vi "Lockin-4461_Multiple Inputs and Outputs_KH_functional_global_waveform_2_2.vi"(8 "stop":bool) -> ()   [LabVIEW 2013]
uses:
  <vilib>/Analysis/4window.llb/windowTd.ctl
  <vilib>/Analysis/3filter.llb/Filter Structure Type.ctl
  <vilib>/Analysis/baseanly.llb/Mean (DBL).vi
  <vilib>/DAQmx/write.llb/DAQmx Write (Analog 1D Wfm NChan NSamp).vi
  <vilib>/Analysis/2dsp.llb/Decimate (single shot).vi
  <vilib>/Analysis/2dsp.llb/Decimate (single shot, DBL).vi
  DAQ-Lockin-SubVI/Lock-in Globles Multiple Inputs and Outputs used with FGV.vi
  <vilib>/Utility/error.llb/Error Cluster From Error Code.vi
  <vilib>/DAQmx/miscellaneous.llb/DAQmx Fill In Error Info.vi
  <vilib>/measure/macond.llb/IIR Filter for N Chan.vi
  <vilib>/measure/maspectr.llb/FFT Power Spectrum and PSD for N Chan.vi
  <vilib>/Analysis/NI_AALBase.lvlib
  <vilib>/measure/NI_MAPro.lvlib
  <vilib>/measure/NI_MABase.lvlib
  <vilib>/Analysis/NI_AALPro.lvlib
panel:
  in  "IIR filter specifications":T1={"Topology"=enum."Butterworth", "Type"=enum."Lowpass", "Order"=1, "Lower Fc"=100.0, "Upper Fc"=200.0, "PB Ripple"=1.0, "SB Attenuation"=60.0} {"PB Ripple" format="%0.2f"; "SB Attenuation" format="%0.2f"; "Lower Fc" format="%0.2p"; "Upper Fc" format="%0.2p"}
  in  "Input Signals":i16(slide)=2 scale=1.0..20.0
  out "phase log":dbl[](array[numeric])=[0.0, 0.0, 0.0, 0.0, 0.0, 6.661338147750939e-16, 0.0, 1.9984014443252818e-15]
  in  "Tab Control 2":T2(tab)=enum."Lock-in Settings"
  in  "Auto control  max AI rate/ AI block size":bool=TRUE
  in  "AI Buffer Size (S)":i32=10
  in  "AI Block Size":i32=1000
  in  "AI Configuration":T3(array[cluster])=[{"AI.Coupling"=10050, "AI.Max"=10.0, "AI.Min"=-10.0, "Input physical channels"="PXI1Slot2/ai0:1"}, {"AI.Coupling"=10050, "AI.Max"=10.0, "AI.Min"=-10.0, "Input physical channels"="PXI1Slot3/ai0:1"}, {"AI.Coupling"=10050, "AI.Max"=10.0, "AI.Min"=-10.0, "Input physical channels"="PXI1Slot5/ai0:1"}, {"AI.Coupling"=10050, "AI.Max"=10.0, "AI.Min"=-10.0, "Input physical channels"="PXI1Slot6/ai0:1"}] {"AI.Coupling" items=["AC"=10045, "DC"=10050, "GND"=10066]}
  in  "AO Configuration":T4(array[cluster])=[{"Output physical channels"="PXI1Slot2/ao0:1", "AO. Max"=0.1, "AO.Min"=-0.1}, {"Output physical channels"="PXI1Slot3/ao0:1", "AO. Max"=0.25, "AO.Min"=-0.25}, {"Output physical channels"="PXI1Slot5/ao0:1", "AO. Max"=0.1, "AO.Min"=-0.1}, {"Output physical channels"="PXI1Slot6/ao0:1", "AO. Max"=0.1, "AO.Min"=-0.1}]
  in  "OSC Configuration":T5(array[cluster])=[[{"Signal Type"=enum."Sine Wave", "DC"=0.0, "Amplitude"=0.01, "frequency"=13.0, "Phase"=0.0}, {"Signal Type"=enum."Sine Wave", "DC"=0.0, "Amplitude"=0.0, "frequency"=13.0, "Phase"=0.0}], [{"Signal Type"=enum."Sine Wave", "DC"=0.0, "Amplitude"=0.0, "frequency"=13.0, "Phase"=0.0}, {"Signal Type"=enum."Sine Wave", "DC"=0.0, "Amplitude"=0.0, "frequency"=13.0, "Phase"=0.0}], [{"Signal Type"=enum."Sine Wave", "DC"=0.0, "Amplitude"=0.0, "frequency"=13.0, "Phase"=0.0}, {"Signal Type"=enum."Sine Wave", "DC"=0.0, "Amplitude"=0.0, "frequency"=13.0, "Phase"=0.0}], [{"Signal Type"=enum."Sine Wave", "DC"=0.0, "Amplitude"=0.0, "frequency"=13.0, "Phase"=0.0}, {"Signal Type"=enum."Sine Wave", "DC"=0.0, "Amplitude"=0.0, "frequency"=13.0, "Phase"=0.0}]] {"frequency" step=0.001 format="%.3p"; "Amplitude" format="%0.2p"; "DC" min=-0.99 max=0.99 format="%.2p"}
  in  "Phase&Tc":T6(array[cluster])=[{"Phase"=0.0, "Time constant"=0.5, "Set Tc"=FALSE, "Autophase"=FALSE, "Order"=0.0}, {"Phase"=0.0, "Time constant"=0.5, "Set Tc"=FALSE, "Autophase"=FALSE, "Order"=0.0}, {"Phase"=0.0, "Time constant"=0.5, "Set Tc"=FALSE, "Autophase"=FALSE, "Order"=0.0}, {"Phase"=0.0, "Time constant"=0.5, "Set Tc"=FALSE, "Autophase"=FALSE, "Order"=0.0}, {"Phase"=0.0, "Time constant"=0.5, "Set Tc"=FALSE, "Autophase"=FALSE, "Order"=0.0}, {"Phase"=0.0, "Time constant"=0.5, "Set Tc"=FALSE, "Autophase"=FALSE, "Order"=0.0}, {"Phase"=0.0, "Time constant"=0.5, "Set Tc"=FALSE, "Autophase"=FALSE, "Order"=0.0}, {"Phase"=0.0, "Time constant"=0.5, "Set Tc"=FALSE, "Autophase"=FALSE, "Order"=0.0}] {"Phase" min=0.0 max=360.0 scale=0.0..360.0}
  in  "Gain":dbl[](array[numeric])=[50000000.0, 50000000.0, 1.0, 1.0, 1.0, 1.0, 1.0, 1.0]
  in  "frequency":dbl=13.0
  out "max ai rate":i32=13000
  out "elapsed time":dbl=138.0
  in  "zero offset":bool
  in  "measure offset":bool
  in  "sample clock multiple (x*f)":i32=1000
  out "AI Rate":dbl=13000.0 format="%.2f"
  out "Display 2":string="-423.350804      n"
  out "Display 1":string="-104.244723      n"
  in  "Remote":bool
  in  "Display":u16(ring) items=["X and Y", "R and Theta"]
  out "Backlog":u8(slide) scale=0.0..100.0
  out "Sampling information":cluster{"Fs":dbl, "#s":dbl}[](array[cluster])=[{"Fs"=13000.0, "#s"=1000.0}]
  out "AO Task":refnum<k21>[](array[refnum])
  out "AI task":refnum<k21>[](array[refnum])
  in  "Tab Control":T7(tab)=enum."Input signals"
  out "Display X (or R) A":dbl[](graph)=[-6.767704118237299e-07, 1.3679095941982762e-06, -8.292119972514093e-07, 1.6081112063430916e-06, -6.48302849428553e-07, 3.3000787620994813e-07, 2.1826626593165523e-07, -4.843594448984296e-07, 7.025229913353154e-07, -4.940803961923873e-07, 5.735003337473624e-07, -3.4668515755027405e-07, -2.4248283537339965e-07, -1.8363287469697745e-08, -3.4589425846339534e-07, 4.6284358832454705e-07, -2.6962179655822256e-07, -1.429402751088828e-07, 9.446578651191532e-08, -5.710117984178673e-09, -5.29242574030563e-07, -7.215176081254315e-08, 2.677231693663559e-07, -2.9474346178622007e-07, 1.6859037233620488e-07, -2.782624102402718e-07, -1.9986912438858682e-07, -3.269593679273288e-08, -2.486510407656373e-07, 5.548402109992747e-07, 9.996987486709427e-08, -6.0130416412624e-08, 9.415818662231201e-08, -2.1083634639079388e-07, 4.091053197976716e-07, -1.1752425483839359e-08, -6.151119173511262e-08, 4.276364767795889e-07, 5.672540816315234e-09, 1.9631938693768442e-07, 3.881923939998436e-07, 3.693414665428258e-07, 2.2443312885204412e-07, -1.0424472343376792e-07, -3.281356459413585e-06, 2.853877661113482e-06, -1.6173510513608656e-06, 2.900242509974247e-07, 3.0449767746807755e-07, -9.53094648189971e-07, 1.19768766975668e-06, -1.6300022513090843e-06, 1.2633381081086798e-06, -1.2597657763077924e-06, 1.5181775758183967e-06, -3.2698180448977813e-07, 4.534684182323745e-22, 2.954958383906869e-22, 2.935987294164666e-22, 2.9919274066034985e-22, 2.4866884846013956e-11, 1.571439962444634e-06, 3.5981993954562916e-05, 4.595320866342681e-05, -3.163614064440566e-05, 2.2025345770237146e-05, -1.4783690228833628e-05, 9.027427496250188e-06, -4.373865947312203e-06, 1.2061179513411652e-06, 2.321934449801555e-06, -3.096117951559957e-06, 3.818767600136303e-06, -2.724223846911526e-06, 2.777457898492608e-06, -1.6318104191727555e-06, 8.644446773102741e-07, 5.245164233996108e-07, -9.074912983112755e-07, 1.5809479476204886e-06, -1.191807434600212e-06, 1.1136104668741203e-06, -8.918436045180084e-07, 7.666775683008394e-07, 4.0094363870758105e-07, -5.024016863890059e-07, 6.184199345905923e-07, -4.547811927193765e-07, 8.577352486006216e-07, -3.929716458984687e-07, -9.250952352542821e-08, 1.4464495001439634e-07, 2.987012020098487e-07, -8.395621078021276e-09, -5.946540278253675e-08, 5.015724336232653e-07, -2.2845172399208505e-07, 2.9148694268542234e-07, -3.3585825169289965e-08, 1.5255809451280384e-07, -1.6688588171069325e-07, 2.9208673634758535e-07, 2.1867560915340566e-08, -1.817033331852077e-09, 2.0922044023006386e-07, -2.0089195447457524e-07, -1.6047621413178067e-07, 3.62693951906398e-07, -4.219972565448854e-07, 2.644775088575862e-07, 1.6782279517097728e-07, -4.0780410649598406e-07, -1.4202551172988562e-07, 4.1098274242707864e-08, 4.0982393853747056e-07, -1.0954576241181e-08, -2.000666884411931e-07, 3.419460779804609e-07, -5.831329333541703e-07, 1.607889368959098e-07, 4.7485928317065607e-07, -1.0986820397700458e-07, 4.234349182513178e-07, 7.50799000900104e-09, -2.913745535551743e-07, 5.212516629832497e-07, -3.5679666811606247e-07, 7.185358920930657e-07, 2.28551626188166e-07, 2.984900132189184e-07, 5.567614355159372e-07, -2.700163649574881e-08, 4.647757728519345e-09, -7.827331963284188e-09, -3.16290394262067e-07, 2.2708072760302243e-07, 7.739366205819891e-08, -4.86859103219973e-07, 2.473259207485168e-07, -3.41601067670072e-07, 1.6627441476941349e-07, 8.910868327391612e-08, -4.126919161116403e-08, 5.064621322918384e-07, -7.216585649893412e-08, 1.7360798289963554e-07, 1.9894946958931327e-07, -1.029870892195247e-07, 1.479174782511515e-08, -7.761128801091328e-08, -9.710807258322806e-08, 2.244692789108791e-07, -5.009546674149695e-07, 2.4630441386600876e-07, 3.701090240857261e-07, -4.940910423104556e-07, 6.97823655978583e-07, 5.463396637012674e-08, 3.3460509656657584e-07, 1.1628795209397034e-07, -9.983904012316269e-08, 2.1194575699660896e-07, -1.4284598126625291e-07, -1.6581535570295627e-07, 1.9543419229659077e-07, 6.421246147653625e-08, 3.817631543808754e-07, 3.5099411367530134e-07, 9.599061510866204e-08, 5.115460403448378e-07, -3.189544820970916e-07, 2.0371122850583007e-07, 7.139469677112191e-08, -2.6780725397357064e-08, 1.8207931762268008e-07, -3.99163483902508e-08, 3.5667336283414435e-24, 2.977721146793187e-22, 2.9488566597725565e-22, 2.931805455672584e-22, 2.8533874679319433e-11, 4.4171853288673887e-07, 1.1776020155369053e-05, 4.5492863810876877e-05, 2.9323742019926304e-05, -2.1525943992685573e-05, 6.085028499678217e-06, 3.4517457636324723e-06, -7.402821485273008e-06, 8.023515280656284e-06, -5.743846711537538e-06, 3.3274091105157146e-06, -7.62703220096605e-07, -1.0696366449954687e-06, 2.5134804524775262e-06, -2.6343637407641244e-06, 2.5318619928474184e-06, -1.7306766758057638e-06, 1.44992950833644e-06, 1.4483945167047895e-07]
  out "Display Y (or Theta) A":dbl[](graph)=[4.765499299686936e-07, -9.658586916637982e-07, -7.621778309143253e-08, -1.5258147249425879e-07, -2.4990753387284357e-07, 1.3419411932204113e-07, -8.565299692875945e-07, 5.571108791407577e-07, -7.860547079397809e-08, -7.196286228942718e-07, 3.4315278763967647e-07, -6.204384175643328e-07, 1.774316085303007e-07, 1.375503590545208e-07, -9.027207823009459e-07, 4.7108028753992357e-07, -1.4273262355224388e-07, -5.084378639622054e-07, 2.0064639544519283e-07, -6.100241361118937e-07, 3.5508186140312606e-07, 1.6599492404614552e-07, -1.1241242632694126e-06, 3.545737663988187e-07, -1.3680834360003273e-07, -5.671646797482132e-07, 3.003111466009731e-07, -7.790822713575479e-07, 3.293880422749827e-07, 3.28274379240407e-08, -1.0651740914596076e-06, 4.2770794764999845e-07, -5.104224380786051e-07, -2.472151922016114e-07, 1.9800282516829894e-07, -7.284254119168647e-07, 5.863115303219669e-07, -2.81773970579004e-07, -7.156335675351997e-07, 2.3981773570157667e-07, -3.978801443495009e-07, 3.035512690481674e-07, -1.7158995838277135e-07, -4.233508035480193e-07, -8.088850970477616e-07, 6.737027936126898e-07, -1.759072178658265e-07, -6.972834404887968e-07, 1.272488135816818e-06, -1.2086621076536852e-06, 4.69525474705048e-07, -4.919175010780031e-08, -3.50864282590232e-07, 6.020350472256037e-07, -9.484640076506137e-07, -6.830224693863262e-08, 1.0170935534147539e-22, -8.29623972830081e-22, -8.014563293027786e-22, -8.094000243152346e-22, 1.3353078985706605e-11, 1.6373548472325611e-07, 1.4866311767580978e-06, -2.707411790797605e-06, 6.830995141435044e-07, -3.8763934216822793e-07, -3.894235373830128e-07, -9.303274404957174e-08, -1.5541472171160917e-07, -1.0548850159824638e-06, 1.301686262269789e-06, -1.9557074574821375e-06, 9.368644690210887e-07, -5.392324932206546e-07, -1.0317815283114626e-06, 9.503284335604831e-07, -1.1138402195810916e-06, -8.612001299094237e-08, 3.392287632745269e-07, -9.880574731396456e-07, 6.176942647460194e-07, -5.670403477561947e-07, -7.529082791811021e-08, 3.797538713075729e-07, -6.875418705429333e-07, 3.774689030428864e-08, 4.010310610815791e-07, -5.552428738314573e-07, 3.8499536868861883e-07, -6.445873434134007e-07, -3.326615731244241e-07, 4.502182873700019e-07, -7.750874192225206e-07, 4.117923202917222e-07, -6.431352998299419e-07, 3.5044644716276235e-07, -1.4225277208615523e-07, -6.876478797176894e-07, 5.399420578514256e-07, -4.5606838526251626e-07, -1.2810883746936567e-07, 7.507205080273586e-07, -1.4012460201934012e-06, 3.6687827494239255e-07, -2.4916075902104696e-07, -6.048091008906423e-07, 6.617540494081048e-07, -1.017139965154715e-06, 6.302573641557335e-07, 4.555496901851896e-07, -1.3339391648309178e-06, 6.715666266662573e-07, -3.8798990954152797e-07, -3.6012440675569084e-07, 5.414910168700109e-07, -1.3243576755919245e-06, 5.902559482413635e-07, -7.542190392147796e-08, -1.0785352133753382e-06, 9.869413956855774e-07, -9.442478036537707e-07, -4.8555902344221593e-08, 5.874045024703844e-07, -1.1585692990263365e-06, 1.3486079750496373e-06, -5.071584526584705e-07, -5.100916917445276e-07, 6.330937674492109e-07, -1.235592399497452e-06, 9.223862720486185e-07, 6.04251856246877e-08, -1.2764854943402043e-06, 8.83547168218078e-07, -9.047288617993288e-07, 2.0116909352114474e-07, 5.358138396845644e-07, -1.3168565866224215e-06, 4.095307061714363e-07, -6.27867381040266e-07, -4.472555022141913e-07, 8.124683056348434e-07, -6.96815296189946e-07, -1.3075261738966236e-07, -2.448175089906454e-07, -3.31091978464826e-07, 4.938406467055916e-07, -1.0121928097926847e-06, 2.6683471402237015e-07, -3.854622779756573e-07, -6.116229848120615e-07, 7.413846592203119e-07, -3.878576789341664e-07, -4.803212369821987e-09, -1.512740254582647e-07, -9.37733298786493e-07, 3.083451264193004e-07, -7.278473080315107e-07, -2.1621978373244913e-07, 1.1649243053043013e-06, -1.5574296555740364e-06, 2.0216029416288657e-07, -1.738290377715283e-08, -8.124252331847678e-07, 8.556517228357048e-07, -1.1895268912765046e-06, -1.6299284686030149e-07, 5.025591222770188e-07, -1.256876728303257e-06, 4.966801881381768e-07, -2.653578297740131e-07, -7.841925208481243e-07, 6.961355949365849e-07, -1.3545884441334733e-06, 1.8978106285789698e-07, -3.1292466455277164e-07, -1.116079741754174e-06, 6.606025379921262e-24, -7.987352443116322e-22, -8.305769155450611e-22, -8.014315043874178e-22, 1.528632786785048e-11, 5.851716352372578e-08, 7.012774926585611e-07, 7.260202605191567e-07, -1.8385722657507987e-06, -7.48491270371179e-07, 1.078630704871155e-06, -5.895807456908318e-07, 1.4658536078852006e-07, 1.0975439156015532e-07, -4.165723785464372e-07, -6.413089995227893e-08, 2.3302809137460278e-07, -4.5082625792713e-08, 1.8812524970362413e-07, 1.2661990176118822e-08, -9.607065782256097e-07, 4.267709983481109e-07, -7.948677906464168e-08, -2.6388811975329723e-07]
  out "Waveform Graph":waveform(dbl)[](graph)
  in  "decimating factor":i32=1
  in  "filter structure option":T8=10 items=["IIR 2nd Order"=0, "IIR 4th Order"=1, "Auto Select"=10]
  out "Waveform Graph 2":cluster{"f0":dbl, "df":dbl, "magnitude":dbl[]}[](graph)
  in  "window":T9=1 items=["Rectangle"=0, "Hanning"=1, "Hamming"=2, "Blackman-Harris"=3, "Exact Blackman"=4, "Blackman"=5, "Flat Top"=6, "4 Term B-Harris "=7, "7 Term B-Harris"=8, "Low Sidelobe"=9, "Blackman Nuttall"=11, "Triangle"=30, "Bartlett-Hanning"=31, "Bohman"=32, "Parzen"=33, "Welch"=34, "Kaiser"=60, "Dolph-Chebyshev"=61, "Gaussian"=62]
  in  "averaging parameters":T10={"averaging mode"=enum."No averaging", "weighting mode"=enum."Exponential", "number of averages"=10} {"number of averages" min=1}
  in  "dB On (F)":bool
  out "Results (X, Y, R, Theta)":dbl[][](array[numeric])=[[-8.990938951699043e-08, -5.496874633933286e-07, 5.569919260950825e-07, -99.28930194172699], [-1.0424472343376792e-07, -4.233508035480193e-07, 4.3599640506377615e-07, -103.83315475232594], [-8.663279130692378e-08, -2.555950511771059e-07, 2.6987788111636043e-07, -108.72385784210852], [-3.572835649086049e-08, -7.56786271488616e-08, 8.368853006639814e-08, -115.2722910768039], [4.431812686724637e-08, 8.517364090161592e-08, 9.601377751895176e-08, 62.51083208252897], [1.4523643643592666e-07, 1.9896598237318188e-07, 2.4633530930488284e-07, 53.87219602328508]] format="%#_6p"
  out "Measure?":u16[](array[numeric])
  in  "Cluster (unused right now)":T11={"Amplitude"=[0.001, 2e-08, 0.001, 0.001, 0.001, 2e-08], "DC"=[0.001, 2e-08, 0.001, 0.001, 0.001, 2e-08], "phase"=[0.001, 2e-08, 0.001, 0.001, 0.001, 2e-08], "Array"=[]}
  out "offsets":dbl[](array[numeric])
  out "Waveform Chart":cluster{dbl, "Numeric":dbl}(graph)
  in  "Rolling Avg Parameters":T12={"Rolling Avg mode"=enum."No Averaging", "# of averages"=10} {"# of averages" min=1}
  in  "index (row)":i32
  in  "disabled index (col)":i32
  # "*****Customized for 4461 + 4462 cards; functional globals*****"
  # "Real time Adjustable Values"
  # "WAVEFORM 2"
  # "Configurations"
  # "should this be x multiple\nof the frequency?"
  # "The top array index selects which card you are setting the outputs for,and the second index selects which output chanel on that card.\n\nFor Phase&Tc, you must have an array element initialized for each input signal."
  # "Features:\n1, Any number of input and output channels\n2, Each AO outputs an DC+AC signal, DC for sample biasing and AC for OSC. These values can be adjusted in real time.\n3, Synchronous filtering\n\nInstructions:\n1, Array index of AI configuration and AO configuration refers to task.\n2, Array index in Amplifier Settings, Phase$&Tc control , and gains correlates to channel number.\n3, Each 4461 board can have 2 lock-in channels. Syntax for 2 channles, e.g. PXI1Slot2/ai0:1. If you want to use just one, then PXI1Slot2/ai0.\n4, Parameters (especially DC value for sample biasing) can be remotely controlled by clicking \"local\"and \"remote\" button. In real experiments, put golable values (can be found in Lock-in globles.vi) in your VI to control the lock-in and read out.\n5, choose OSC frequencies to be multiple of \nAI Rate/AI Block SIze to have best performance.\n\n-Guanglei 06/23/2011\n\nUpdate:\n1. Allows any number of lockin amplifiers and AO tasks.\n2. Delete the channels from any AI/AO Configuration elements you do not want to use.\n3. Rows (first index) of the OSC Configuration correspond to different AO tasks, while columns (second index) correspond to AO channels in that task. All channels in a given element of the AO Configuration array will go into a single task.\n4. The same number of output channels must go in each AO task.\n5. Make sure a Phase&Tc element and an Amplifier Settings element is set for each AI channel.\n-Joe 12/3/2013"
  # "hide stuff here in this tab"
  # "multiple of frequency??"
  # "this is \"time constant\""
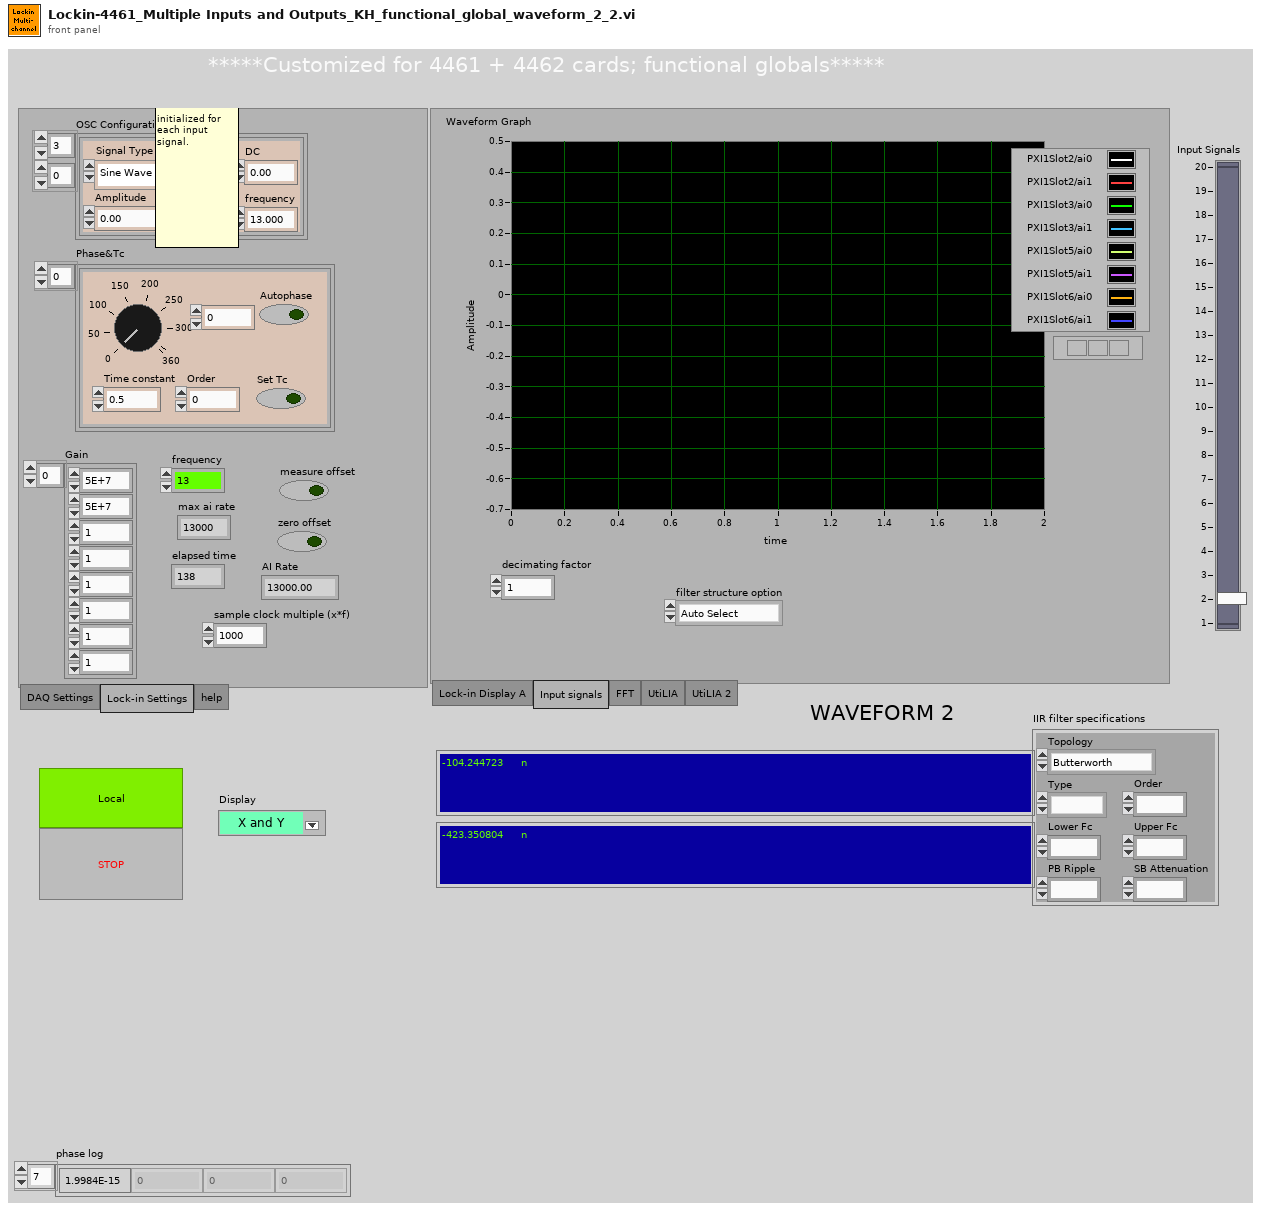
[diagram p1: front panel]
types:
  T1 = cluster{"Topology":enum16{"Off", "Butterworth", "Chebyshev", "Inverse Chebyshev", "Elliptic", "Bessel"}, "Type":enum16{"Lowpass", "Highpass", "Bandpass", "Bandstop"}, "Order":i32, "Lower Fc":dbl, "Upper Fc":dbl, "PB Ripple":dbl, "SB Attenuation":dbl}
  T2 = enum32{"DAQ Settings", "Lock-in Settings", "help"}
  T3 = cluster{"AI.Coupling":i32, "AI.Max":dbl, "AI.Min":dbl, "Input physical channels":tag}[]
  T4 = cluster{"Output physical channels":tag, "AO. Max":dbl, "AO.Min":dbl}[]
  T5 = cluster{"Signal Type":enum16{"Sine Wave", "Triangle Wave", "Square Wave", "Sawtooth Wave"}, "DC":dbl, "Amplitude":dbl, "frequency":dbl, "Phase":dbl}[][]
  T6 = cluster{"Phase":dbl, "Time constant":dbl, "Set Tc":bool, "Autophase":bool, "Order":dbl}[]
  T7 = enum32{"Lock-in Display A", "Input signals", "FFT", "UtiLIA", "UtiLIA 2"}
  T8 = typedef "NI_AALBase.lvlib/Filter Structure Type.ctl" = u16
  T9 = typedef "NI_AALPro.lvlib/windowTd.ctl" = u32
  T10 = cluster{"averaging mode":enum16{"No averaging", "Vector averaging", "RMS averaging", "Peak hold"}, "weighting mode":enum16{"Linear", "Exponential"}, "number of averages":u32}
  T11 = cluster{"Amplitude":dbl[], "DC":dbl[], "phase":dbl[], "Array":enum16{"Sine Wave", "Triangle Wave", "Square Wave", "Sawtooth Wave"}[]}
  T12 = cluster{"Rolling Avg mode":enum16{"No Averaging", "Linear", "Exponential"}, "# of averages":u32}
  T13 = cluster{"Signal Type":enum16{"Sine Wave", "Triangle Wave", "Square Wave", "Sawtooth Wave"}, "DC":dbl, "Amplitude":dbl, "frequency":dbl, "Phase":dbl}
  T14 = cluster{"Chunk Average":dbl, "Long-term Average":dbl}
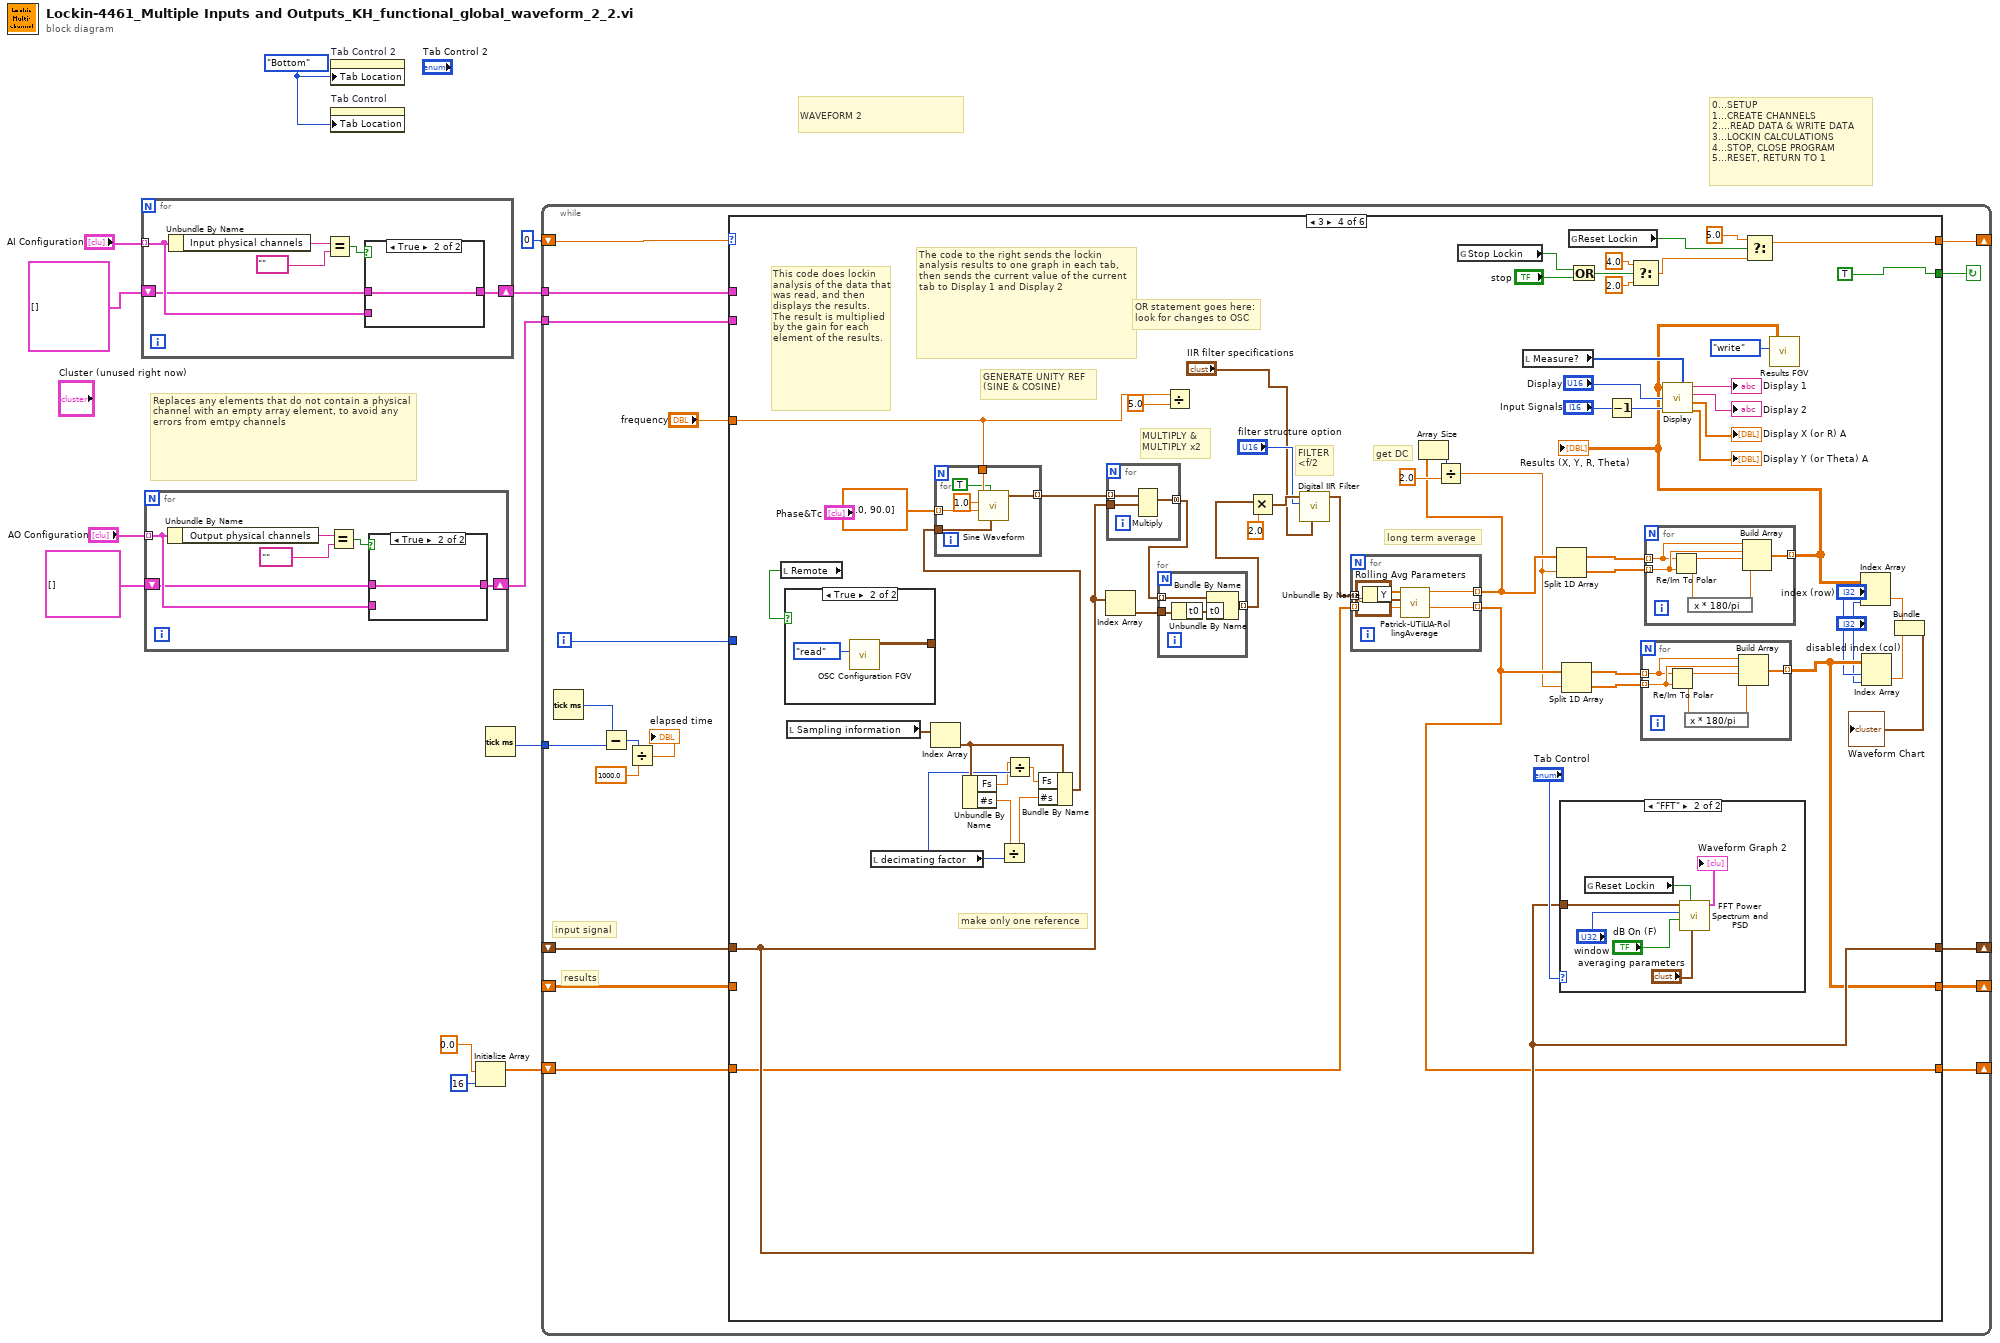
[diagram p0: block diagram]
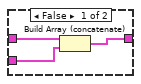
[diagram p2: hidden frame]
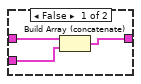
[diagram p3: hidden frame]
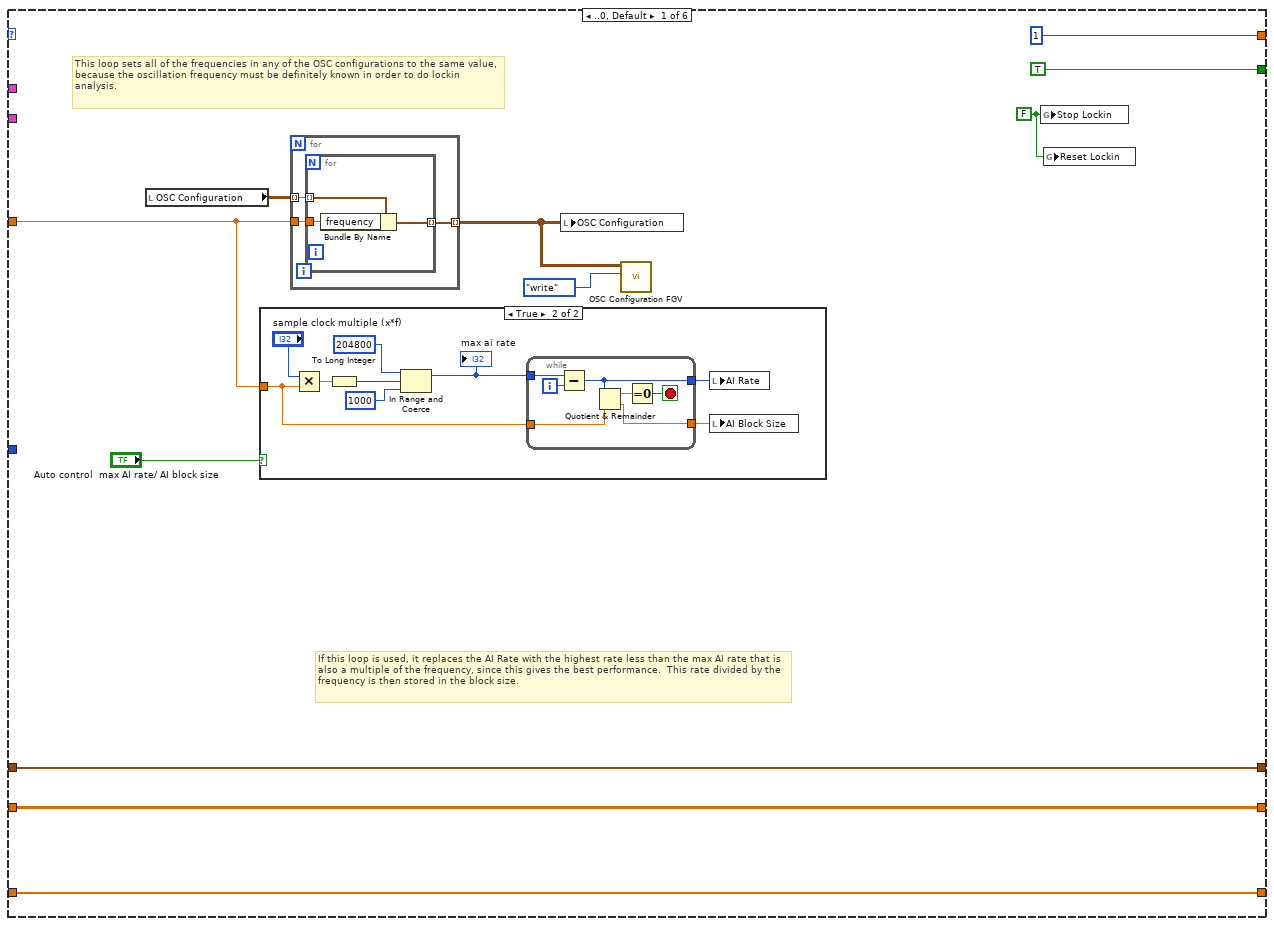
[diagram p4: hidden frame]
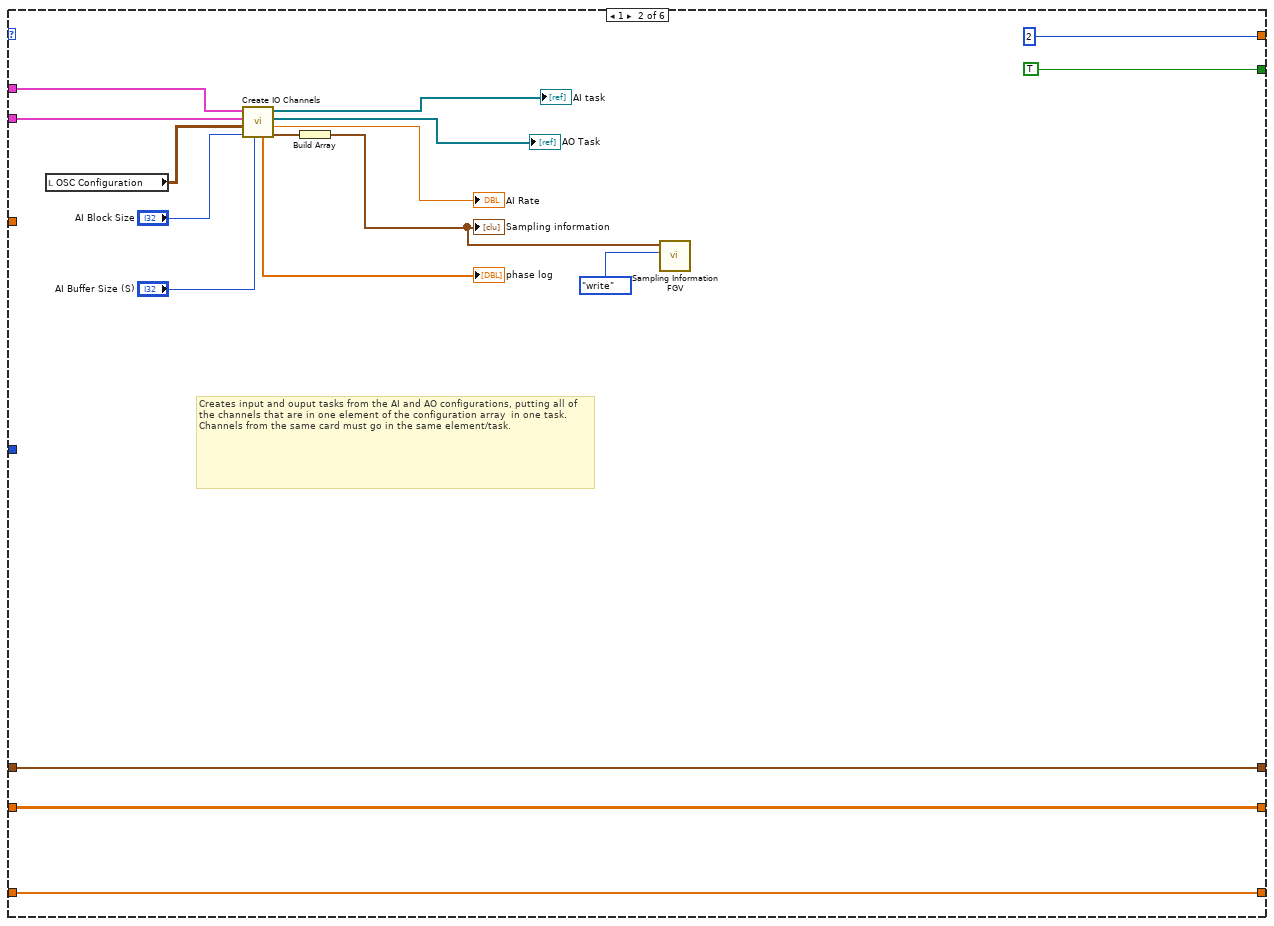
[diagram p6: hidden frame]
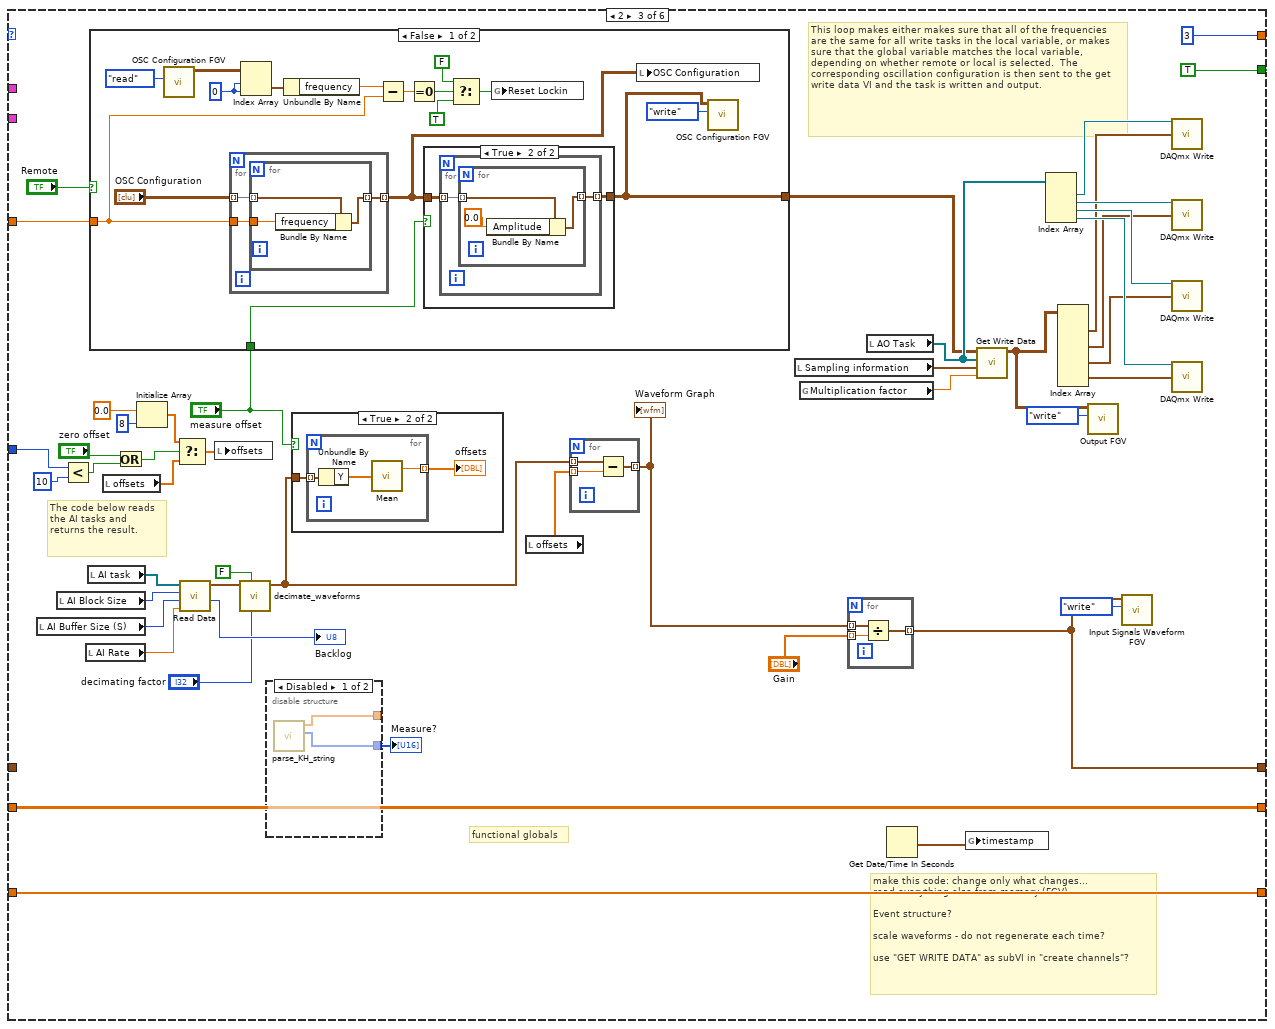
[diagram p7: hidden frame]
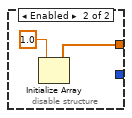
[diagram p9: hidden frame]
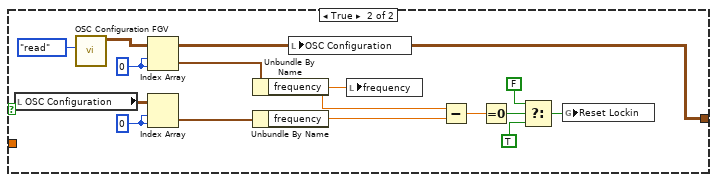
[diagram p11: hidden frame]
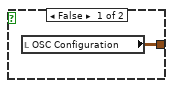
[diagram p13: hidden frame]
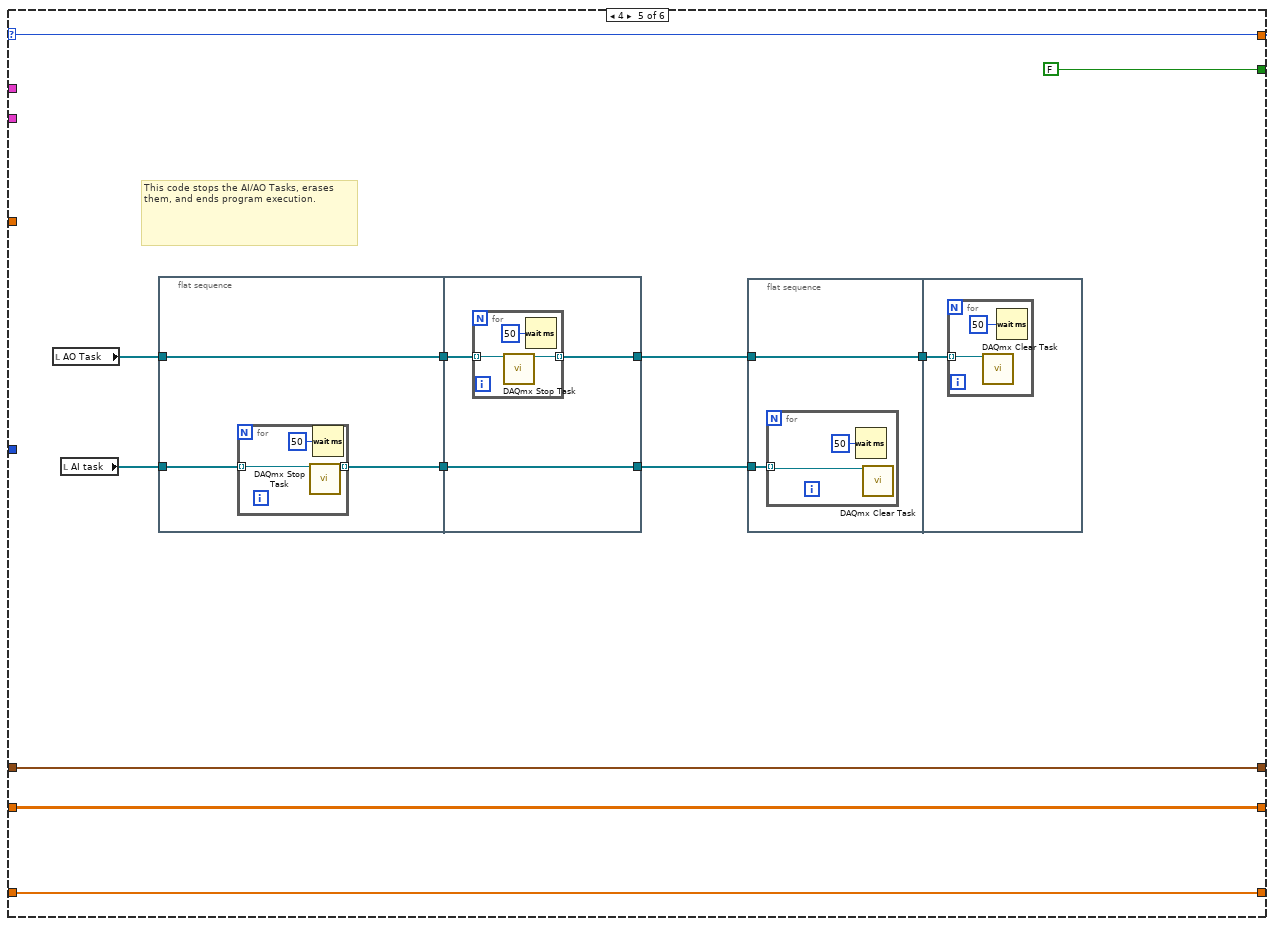
[diagram p14: hidden frame]
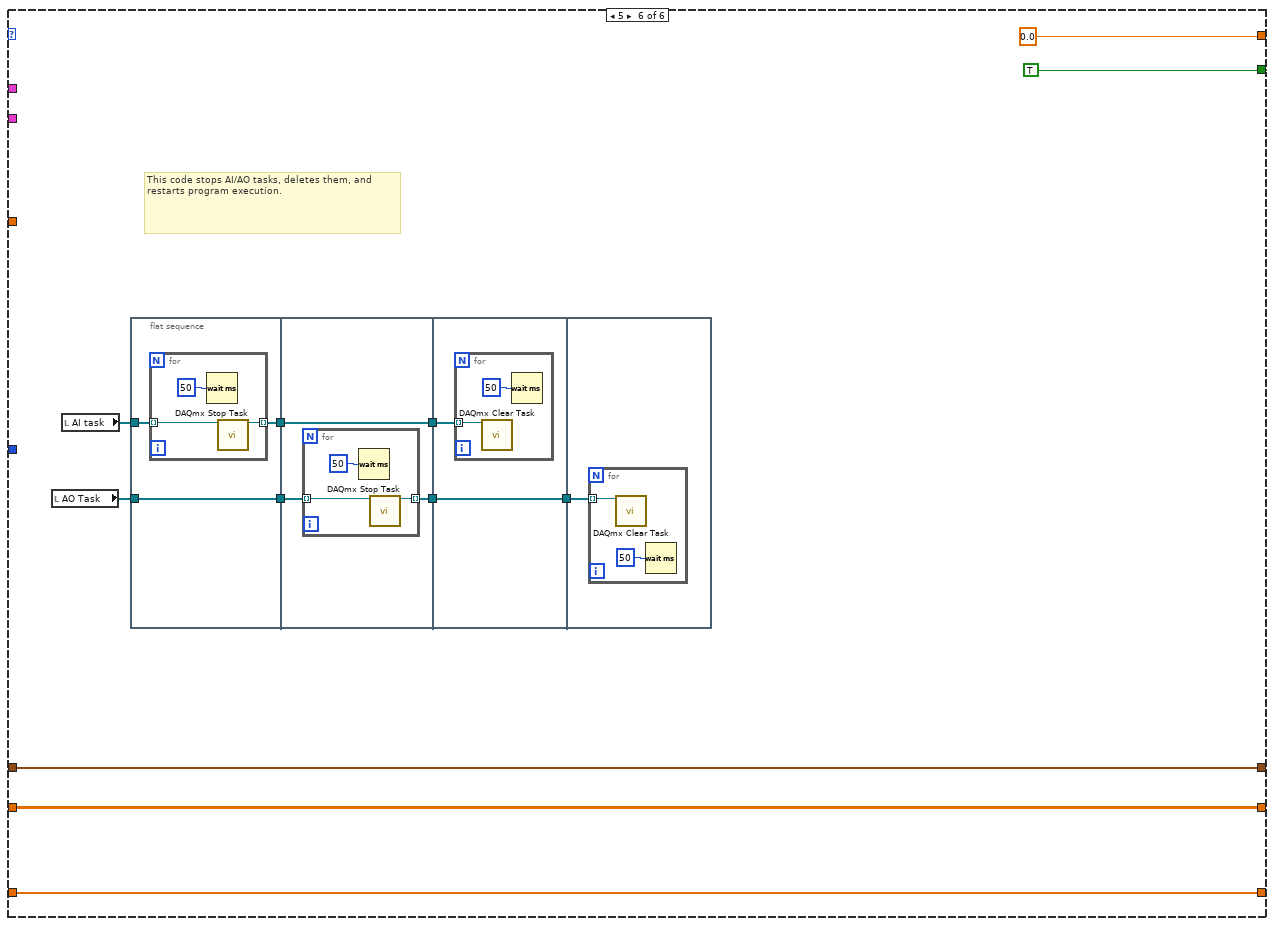
[diagram p15: hidden frame]
diagram:
  w7 = enum32{"Top", "Bottom", "Left", "Right"}."Bottom" ("Tab Location")
  # "0...SETUP\n1...CREATE CHANNELS\n2....READ DATA & WRITE DATA\n3...LOCKIN CALCULATIONS\n4...STOP, CLOSE PROGRAM\n5...RESET, RETURN TO 1"
  # "WAVEFORM 2"
  # "Replaces any elements that do not contain a physical channel with an empty array element, to avoid any errors from emtpy channels"
  n1 = for {
    tunnel: "AI Configuration" -> [w15] mode=indexing
    shift-right: [w13] -> w12
    shift-left: T3 [] ("AI Configuration") -> [w14]
    n2 = Unbundle By Name(w15) -> ("Input physical channels"=w17:tag)
    n3 = Equal?(x=w17, y=tag "" ("Empty physical channels")) -> (x = y?=w18:bool)
    n4 = case shown="True" w18 {
      tunnel: w15 -> [w20 _]
      tunnel: w14 -> [w21 w22]
      tunnel: [w19 w22] -> w13
      frame False {
        n5 = Build Array (concatenate)(w21, w20) -> (w19:T3)
      }
      frame True {
      }
    }
  }
  n6 = for {
    tunnel: "AO Configuration" -> [w25] mode=indexing
    shift-right: [w23] -> w5
    shift-left: T4 [] ("AO Configuration 2") -> [w24]
    n7 = Unbundle By Name(w25) -> ("Output physical channels"=w27:tag)
    n8 = Equal?(x=w27, y=tag "" ("Empty physical channels")) -> (x = y?=w28:bool)
    n9 = case shown="True" w28 {
      tunnel: w25 -> [w30 _]
      tunnel: w24 -> [w31 w32]
      tunnel: [w29 w32] -> w23
      frame False {
        n10 = Build Array (concatenate)(w31, w30) -> (w29:T4)
      }
      frame True {
      }
    }
  }
  n11 = property on="Tab Control 2" class="TabCtl (strict)"("Tab Location"=w7) -> ()  [unwired: 2 in, 2 out]
  n12 = property on="Tab Control" class="TabCtl (strict)"("Tab Location"=w7) -> ()  [unwired: 2 in, 2 out]
  n13 = Initialize Array(0.0, 16 ("dimension size")) -> (w3:dbl[])
  n14 = Tick Count (ms)() -> (millisecond timer value=w1:u32)
  n15 = while {
    shift-right: [w50] -> _
    shift-left: 0 -> [w49]
    tunnel: w12 -> [w48]
    tunnel: w5 -> [w46]
    shift-right: [w45] -> _
    shift-left: _ -> [w44]
    shift-right: [w42] -> _
    shift-left: _ -> [w43]
    shift-right: [w40] -> _
    shift-left: w3 -> [w39]
    tunnel: w1 -> [w36]
    i -> [w41]
    stop <- w47 continue-if-true
    # "results"
    # "input signal"
    n16 = Tick Count (ms)() -> (millisecond timer value=w37:u32)
    n17 = Subtract(x=w37, y=w36) -> (x-y=w35:u32)
    n18 = Divide(x=w35, y=1000.0) -> (x/y=→"elapsed time":dbl)
    n19 = case shown="3" w49 {
      selector: w49 -> [_ _ _ _ w316 _]
      tunnel: [1 2 3 w257 w316 0.0 ("f")] -> w50
      tunnel: w48 -> [_ w95 _ _ _ _]
      tunnel: [TRUE TRUE TRUE TRUE FALSE TRUE] -> w47
      tunnel: w46 -> [_ w94 _ _ _ _]
      tunnel: [w54 w89 w122 w223 w308 w339] -> w45
      tunnel: w44 -> [w54 w89 _ w223 w308 w339]
      tunnel: w43 -> [w53 w88 w137 _ w307 w338]
      tunnel: [w53 w88 w137 w221 w307 w338] -> w42
      tunnel: w41 -> [_ _ w132 _ _ _]
      tunnel: [w52 w85 w135 w211 w306 w337] -> w40
      tunnel: w39 -> [w52 w85 w135 w210 w306 w337]
      tunnel: "frequency" -> [w51 _ w134 w237 _ _]
      frame ..0, Default {
        w60 = FALSE ("Stop Lockin")
        # "If this loop is used, it replaces the AI Rate with the highest rate less than the max AI rate that is also a multiple of the frequency, since this gives the best performance.  This rate divided by the frequency is then stored in the block size."
        # "This loop sets all of the frequencies in any of the OSC configurations to the same value, because the oscillation frequency must be definitely known in order to do lockin analysis."
        n20 = local read "OSC Configuration"() -> (w57:T5)
        n21 = case shown="True" "Auto control  max AI rate/ AI block size" {
          tunnel: w51 -> [_ w68]
          frame False {
          }
          frame True {
            n22 = Multiply(x="sample clock multiple (x*f)", y=w68) -> (x*y=w74:dbl)
            n23 = To Long Integer(number=w74) -> (32bit integer=w72:i32)
            n24 = In Range and Coerce(upper limit=204800, x=w72, lower limit=1000) -> (coerced(x)=w69:i32)  [unwired: 1 out]
            "max ai rate" <- w69
            n25 = while {
              tunnel: w69 -> [w83]
              tunnel: [w81] -> w76
              tunnel: [w79] -> w75
              tunnel: w68 -> [w80]
              i -> [w82]
              stop <- w77 stop-if-true
              n26 = Subtract(x=w83, y=w82) -> (x-y=w79:i32)
              n27 = Quotient & Remainder(x=w79, y=w80) -> (x-y*floor(x/y)=w78:dbl, floor(x/y)=w81:dbl)
              n28 = Equal To 0?(x=w78) -> (x = 0?=w77:bool)
            }
            n29 = local write "AI Rate"(w75) -> ()
            n30 = local write "AI Block Size"(w76) -> ()
          }
        }
        n31 = for {
          tunnel: w57 -> [w64] mode=indexing
          tunnel: [w63] -> w56 mode=indexing
          tunnel: w51 -> [w62]
          n32 = for {
            tunnel: w64 -> [w67] mode=indexing
            tunnel: [w66] -> w63 mode=indexing
            tunnel: w62 -> [w65]
            n33 = Bundle By Name(cluster=w67, "frequency"=w65) -> (w66:T13)
          }
        }
        n34 = local write "OSC Configuration"(w56) -> ()
        n35 = call "OSC Configuration FGV.vi"("Function"=enum16{"write", "read"}."write", "OSC Configuration"=w56) -> ()  [unwired: 4 in, 2 out]
        n36 = global write "Lock-in Globles Multiple Inputs and Outputs used with FGV.vi" "Stop Lockin"(w60) -> ()
        n37 = global write "Lock-in Globles Multiple Inputs and Outputs used with FGV.vi" "Reset Lockin"(w60) -> ()
      }
      frame 1 {
        # "Creates input and ouput tasks from the AI and AO configurations, putting all of the channels that are in one element of the configuration array  in one task.  Channels from the same card must go in the same element/task."
        n38 = local read "OSC Configuration"() -> (w98:T5)
        n39 = call "Create IO Channels.vi"("AI Buffer Size (s)"="AI Buffer Size (S)", "AI Block Size"="AI Block Size", "OSC Configuration"=w98, "AO Configuration"=w94, "AI Configuration"=w95) -> ("sampling info"=w90:cluster{"Fs":dbl, "#s":dbl}, "AI Rate"=→"AI Rate":dbl, "AO Task"=→"AO Task":refnum<k21>[], "AI task"=→"AI task":refnum<k21>[], "phase log"=→"phase log":dbl[])  [unwired: 1 in, 1 out]
        n40 = Build Array(w90) -> (w84:cluster{"Fs":dbl, "#s":dbl}[])
        "Sampling information" <- w84
        n41 = call "Sampling Information FGV.vi"("Function"=enum16{"write", "read"}."write", "Sampling information"=w84) -> ()  [unwired: 4 in, 2 out]
      }
      frame 2 {
        # "make this code: change only what changes...\nread everything else from memory (FGV)\n\nEvent structure?\n\nscale waveforms - do not regenerate each time?\n\nuse \"GET WRITE DATA\" as subVI in \"create channels\"?"
        # "functional globals"
        # "The code below reads the AI tasks and returns the result."
        # "This loop makes either makes sure that all of the frequencies are the same for all write tasks in the local variable, or makes sure that the global variable matches the local variable, depending on whether remote or local is selected.  The corresponding oscillation configuration is then sent to the get write data VI and the task is written and output."
        n42 = local read "AI Buffer Size (S)"() -> (w139:i32)
        n43 = local read "AI Block Size"() -> (w140:i32)
        n44 = Less?(x=w132, y=10) -> (x < y?=w125:bool)
        n45 = local read "AI Rate"() -> (w138:dbl)
        n46 = local read "AI task"() -> (w141:refnum<k21>[])
        n47 = case shown="False" "Remote" {
          tunnel: [w163 w193] -> w113
          tunnel: w134 -> [w166 _]
          tunnel: "measure offset" -> [w165 _]
          frame False {
            w175 = 0 ("index")
            n48 = call "OSC Configuration FGV.vi"("Function"=enum16{"write", "read"}."read") -> ("OSC Configuration"=w169:T5)  [unwired: 5 in, 1 out]
            n49 = for {
              tunnel: w166 -> [w189]
              tunnel: "OSC Configuration" -> [w188] mode=indexing
              tunnel: [w187] -> w164 mode=indexing
              n50 = for {
                tunnel: w188 -> [w192] mode=indexing
                tunnel: w189 -> [w191]
                tunnel: [w190] -> w187 mode=indexing
                n51 = Bundle By Name(cluster=w192, "frequency"=w191) -> (w190:T13)
              }
            }
            n52 = Index Array(array=w169, index (row)=w175, index (col)=w175) -> (element=w174:T13)
            n53 = Unbundle By Name(w174) -> ("frequency"=w168:dbl)
            n54 = Subtract(x=w168, y=w166) -> (x-y=w167:dbl)
            n55 = Equal To 0?(x=w167) -> (x = 0?=w173:bool)
            n56 = case shown="True" w165 {
              tunnel: w164 -> [w179 w181]
              tunnel: [w179 w180] -> w163
              frame False {
              }
              frame True {
                n57 = for {
                  tunnel: w181 -> [w183] mode=indexing
                  tunnel: [w182] -> w180 mode=indexing
                  n58 = for {
                    tunnel: w183 -> [w186] mode=indexing
                    tunnel: [w185] -> w182 mode=indexing
                    n59 = Bundle By Name(cluster=w186, "Amplitude"=0.0) -> (w185:T13)
                  }
                }
              }
            }
            n60 = Select(t=FALSE ("Reset Lockin"), s=w173, f=TRUE ("Reset Lockin")) -> (s? t:f=w170:bool)
            n61 = global write "Lock-in Globles Multiple Inputs and Outputs used with FGV.vi" "Reset Lockin"(w170) -> ()
            n62 = local write "OSC Configuration"(w164) -> ()
            n63 = call "OSC Configuration FGV.vi"("Function"=enum16{"write", "read"}."write", "OSC Configuration"=w163) -> ()  [unwired: 4 in, 2 out]
          }
          frame True {
            w203 = 0 ("index")
            w205 = 0 ("index")
            n64 = local read "OSC Configuration"() -> (w195:T5)
            n65 = call "OSC Configuration FGV.vi"("Function"=enum16{"write", "read"}."read") -> ("OSC Configuration"=w193:T5)  [unwired: 5 in, 1 out]
            n66 = Index Array(array=w193, index (row)=w205, index (col)=w205) -> (element=w206:T13)
            n67 = Index Array(array=w195, index (row)=w203, index (col)=w203) -> (element=w202:T13)
            n68 = Unbundle By Name(w206) -> ("frequency"=w194:dbl)
            n69 = Unbundle By Name(w202) -> ("frequency"=w200:dbl)
            n70 = local write "OSC Configuration"(w193) -> ()
            n71 = local write "frequency"(w194) -> ()
            n72 = Subtract(x=w194, y=w200) -> (x-y=w201:dbl)
            n73 = Equal To 0?(x=w201) -> (x = 0?=w199:bool)
            n74 = Select(t=FALSE ("Reset Lockin"), s=w199, f=TRUE ("Reset Lockin")) -> (s? t:f=w196:bool)
            n75 = global write "Lock-in Globles Multiple Inputs and Outputs used with FGV.vi" "Reset Lockin"(w196) -> ()
          }
        }
        n76 = local read "offsets"() -> (w131:dbl[])
        n77 = Or(x="zero offset", y=w125) -> (x .or. y?=w124:bool)
        n78 = Initialize Array(0.0, 8 ("dimension size")) -> (w128:dbl[])
        n79 = Select(t=w128, s=w124, f=w131) -> (s? t:f=w130:dbl[])
        n80 = call "Read Data.vi"("AI Rate"=w138, "AI Buffer Size (s)"=w139, "AI Block Size"=w140, "AI task"=w141) -> ("Backlog"=→"Backlog":u8, "Input Signals"=w119:waveform(dbl)[])  [unwired: 5 in, 1 out]
        n81 = local write "offsets"(w130) -> ()
        n82 = call "decimate_waveforms.vi"("decimating factor"="decimating factor", "averaging"=FALSE, "Input Signal"=w119) -> ("Decimated Waveforms"=w114:waveform(dbl)[])  [unwired: 7 in, 1 out]
        n83 = disable-structure shown="Disabled" {
          disable-tunnel: [w160 w161] -> _
          disable-tunnel: [w159 _] -> w133
          frame Disabled {
            n84 = call "parse_KH_string.vi"() -> ("Measurement type"=w159:i32[], "Gain"=w160:dbl[])  [unwired: 10 in]
          }
          frame Enabled {
            n85 = Initialize Array(1.0) -> (w161:dbl[])  [unwired: 1 in]
          }
        }
        "Measure?" <- w133
        n86 = case shown="True" "measure offset" {
          tunnel: w114 -> [_ w148]
          frame False {
          }
          frame True {
            n87 = for {
              tunnel: [w152] -> w149 mode=indexing
              tunnel: w148 -> [w151] mode=indexing
              n88 = Unbundle By Name(w151) -> ("Y"=w150:dbl[])
              n89 = call-poly <vilib>:"Mean.vi"("X"=w150) -> ("mean"=w152:dbl)  [unwired: 1 out]
            }
            "offsets" <- w149
          }
        }
        n90 = local read "offsets"() -> (w123:dbl[])
        n91 = for {
          tunnel: w114 -> [w155] mode=indexing
          tunnel: [w154] -> w101 mode=indexing
          tunnel: w123 -> [w153] mode=indexing
          n92 = Subtract(x=w155, y=w153) -> (x-y=w154:waveform(dbl))
        }
        "Waveform Graph" <- w101
        n93 = local read "Sampling information"() -> (w143:cluster{"Fs":dbl, "#s":dbl}[])
        n94 = global read "Lock-in Globles Multiple Inputs and Outputs used with FGV.vi" "Multiplication factor"() -> (w142:dbl)
        n95 = for {
          tunnel: w101 -> [w158] mode=indexing
          tunnel: [w157] -> w122 mode=indexing
          tunnel: "Gain" -> [w156] mode=indexing
          n96 = Divide(x=w158, y=w156) -> (x/y=w157:waveform(dbl))
        }
        n97 = local read "AO Task"() -> (w115:refnum<k21>[])
        n98 = Get Date/Time In Seconds() -> (seconds since 1Jan1904=w144:timestamp)
        n99 = global write "Lock-in Globles Multiple Inputs and Outputs used with FGV.vi" "timestamp"(w144) -> ()
        n100 = call "Get Write Data.vi"("Multiplication Factor"=w142, "Sampling information 2"=w143, "AO Task"=w115, "OSC Configuration"=w113) -> ("Data"=w103:waveform(dbl)[][])  [unwired: 7 in]
        n101 = Index Array(array=w115) -> (element #1=w112:refnum<k21>, element #2=w111:refnum<k21>, element #3=w110:refnum<k21>, element #4=w109:refnum<k21>)  [unwired: 4 in]
        n102 = Index Array(array=w103) -> (element #1=w108:waveform(dbl)[], element #2=w107:waveform(dbl)[], element #3=w106:waveform(dbl)[], element #4=w105:waveform(dbl)[])  [unwired: 8 in]
        n103 = call "Output FGV.vi"("Function"=enum16{"write", "read"}."write", "Output"=w103) -> ()  [unwired: 4 in, 2 out]
        n104 = call "Input Signals Waveform FGV.vi"("Function"=enum16{"write", "read"}."write", "input signal"=w122) -> ()  [unwired: 4 in, 2 out]
        n105 = call-poly <vilib>:"DAQmx Write.vi"("task/channels in"=w112, "data"=w108) -> ()  [unwired: 11 in, 3 out]
        n106 = call-poly <vilib>:"DAQmx Write.vi"("task/channels in"=w111, "data"=w107) -> ()  [unwired: 11 in, 3 out]
        n107 = call-poly <vilib>:"DAQmx Write.vi"("task/channels in"=w110, "data"=w106) -> ()  [unwired: 11 in, 3 out]
        n108 = call-poly <vilib>:"DAQmx Write.vi"("task/channels in"=w109, "data"=w105) -> ()  [unwired: 11 in, 3 out]
      }
      frame 3 {
        # "long term average"
        # "get DC"
        # "FILTER\n<f/2"
        # "MULTIPLY &\nMULTIPLY x2"
        # "GENERATE UNITY REF\n(SINE & COSINE)"
        # "make only one reference"
        # "OR statement goes here:\nlook for changes to OSC"
        # "The code to the right sends the lockin analysis results to one graph in each tab, then sends the current value of the current tab to Display 1 and Display 2"
        # "This code does lockin analysis of the data that was read, and then displays the results.  The result is multiplied by the gain for each element of the results."
        n109 = local read "Remote"() -> (w256:bool)
        n110 = case shown="True" w256 {
          tunnel: [w303 w304] -> _
          frame False {
            n111 = local read "OSC Configuration"() -> (w303:T5)
          }
          frame True {
            n112 = call "OSC Configuration FGV.vi"("Function"=enum16{"write", "read"}."read") -> ("OSC Configuration"=w304:T5)  [unwired: 5 in, 1 out]
          }
        }
        n113 = local read "Sampling information"() -> (w249:cluster{"Fs":dbl, "#s":dbl}[])
        n114 = local read "decimating factor"() -> (w231:i32)
        n115 = Index Array(array=w249) -> (element=w235:cluster{"Fs":dbl, "#s":dbl})  [unwired: 1 in]
        n116 = Unbundle By Name(w235) -> ("Fs"=w230:dbl, "#s"=w234:dbl)
        n117 = Divide(x=w234, y=w231) -> (x/y=w233:dbl)
        n118 = Divide(x=w230, y=w231) -> (x/y=w229:dbl)
        n119 = Bundle By Name(cluster=w235, "Fs"=w229, "#s"=w233) -> (w227:cluster{"Fs":dbl, "#s":dbl})
        n120 = for {
          tunnel: w227 -> [w285]
          tunnel: w237 -> [w289]
          tunnel: [w288] -> w232 mode=indexing
          tunnel: dbl[] [0.0, 90.0] -> [w287] mode=indexing
          n121 = call <vilib>:"Sine Waveform.vi"("sampling info"=w285, "reset signal"=TRUE, "phase"=w287, "amplitude"=1.0, "frequency"=w289) -> ("signal out"=w288:waveform(dbl))  [unwired: 5 in, 1 out]
        }
        n122 = Index Array(array=w223) -> (element=w222:waveform(dbl))  [unwired: 1 in]
        n123 = for {
          tunnel: [w282] -> w228 mode=concatenating
          tunnel: w223 -> [w284]
          tunnel: w232 -> [w283] mode=indexing
          n124 = Multiply(1:w284, 2:w283) -> (0:w282:waveform(dbl)[])  [unwired: 1 in, 1 out]
        }
        n125 = for {
          tunnel: w228 -> [w281] mode=indexing
          tunnel: w222 -> [w279]
          tunnel: [w278] -> w226 mode=indexing
          n126 = Unbundle By Name(w279) -> ("t0"=w280:timestamp)
          n127 = Bundle By Name(cluster=w281, "t0"=w280) -> (w278:waveform(dbl))
        }
        n128 = Divide(x=w237, y=5.0) -> ()  [unwired: 1 out]
        n129 = Multiply(x=w226, y=2.0) -> (x*y=w242:waveform(dbl)[])
        n130 = call-poly <vilib>:"Digital IIR Filter.vi"("IIR filter specifications"="IIR filter specifications", "filter structure option"="filter structure option", "signal(s) in"=w242) -> ("signal(s) out"=w215:waveform(dbl)[])  [unwired: 6 in, 2 out]
        n131 = for {
          tunnel: w215 -> [w277] mode=indexing
          tunnel: [w275] -> w212 mode=indexing
          tunnel: [w274] -> w211 mode=indexing
          tunnel: w210 -> [w273] mode=indexing
          n132 = Unbundle By Name(w277) -> ("Y"=w276:dbl[])
          n133 = call "Patrick-UTiLIA-RollingAverage.vi"("Current Average"=w273, "Rolling Avg Parameters"="Rolling Avg Parameters", "Signal to Average"=w276) -> ("Long-term Average"=w274:dbl, "Chunk Average"=w275:dbl)  [unwired: 1 in, 3 out]
        }
        n134 = Array Size(array=w212) -> (size(s)=w241:i32)
        n135 = Divide(x=w241, y=2.0) -> (x/y=w209:dbl)
        n136 = global read "Lock-in Globles Multiple Inputs and Outputs used with FGV.vi" "Stop Lockin"() -> (w262:bool)
        n137 = local read "Measure?"() -> (w245:u16[])
        n138 = Split 1D Array(array=w212, index=w209) -> (first subarray=w225:dbl[], second subarray=w224:dbl[])
        n139 = case shown="\"FFT\"" "Tab Control" {
          tunnel: w223 -> [_ w292]
          frame "Input signals", Default {
          }
          frame "FFT" {
            n140 = global read "Lock-in Globles Multiple Inputs and Outputs used with FGV.vi" "Reset Lockin"() -> (w296:bool)
            n141 = call-poly <vilib>:"FFT Power Spectrum and PSD.vi"("averaging parameters"="averaging parameters", "restart averaging (F)"=w296, "dB On (F)"="dB On (F)", "window"="window", "time signals"=w292) -> ("Power Spectrum / PSD"=→"Waveform Graph 2":cluster{"f0":dbl, "df":dbl, "magnitude":dbl[]}[])  [unwired: 3 in, 3 out]
          }
        }
        n142 = Split 1D Array(array=w211, index=w209) -> (first subarray=w214:dbl[], second subarray=w213:dbl[])
        n143 = global read "Lock-in Globles Multiple Inputs and Outputs used with FGV.vi" "Reset Lockin"() -> (w251:bool)
        n144 = Or(x=w262, y="stop") -> (x .or. y?=w260:bool)
        n145 = Decrement(x="Input Signals") -> (x-1=w253:i16)
        n146 = Select(t=4.0 ("f"), s=w260, f=2.0) -> (s? t:f=w259:dbl)
        n147 = for {
          tunnel: w214 -> [w297] mode=indexing
          tunnel: w213 -> [w299] mode=indexing
          tunnel: [w298] -> w221 mode=indexing
          n148 = Re/Im To Polar(2:w299, 3:w297) -> (0:w302:dbl, 1:w300:dbl)
          n149 = expression code="x * 180/pi"(w302) -> (w301:dbl)
          n150 = Build Array(w297, w299, w300, w301) -> (w298:dbl[])
        }
        n151 = for {
          tunnel: w225 -> [w266] mode=indexing
          tunnel: w224 -> [w268] mode=indexing
          tunnel: [w267] -> w208 mode=indexing
          n152 = Re/Im To Polar(2:w268, 3:w266) -> (0:w271:dbl, 1:w269:dbl)
          n153 = expression code="x * 180/pi"(w271) -> (w270:dbl)
          n154 = Build Array(w266, w268, w269, w270) -> (w267:dbl[])
        }
        "Results (X, Y, R, Theta)" <- w208
        n155 = call "Display.vi"("Results"=w208, "Display"="Display", "Lock-in #"=w253, "Amplifier Settings"=w245) -> ("Display 1"=→"Display 1":string, "Display 2"=→"Display 2":string, "Array"=→"Display X (or R) A":dbl[], "Array 2"=→"Display Y (or Theta) A":dbl[])  [unwired: 3 in]
        n156 = Select(t=5.0, s=w251, f=w259) -> (s? t:f=w257:dbl)
        n157 = call "Results FGV.vi"("Function"=enum16{"write", "read"}."write", "Input Signals"=w208) -> ()  [unwired: 4 in, 2 out]
        n158 = Index Array(array=w208, index (row)="index (row)", index (col)="disabled index (col)") -> (element=w217:dbl)
        n159 = Index Array(array=w221, index (row)="index (row)", index (col)="disabled index (col)") -> (element=w218:dbl)
        n160 = Bundle("Chunk Average"=w217, "Long-term Average"=w218) -> (→"Waveform Chart":T14)  [unwired: 1 in]
      }
      frame 4 {
        # "This code stops the AI/AO Tasks, erases them, and ends program execution."
        n161 = local read "AO Task"() -> (w313:refnum<k21>[])
        n162 = local read "AI task"() -> (w315:refnum<k21>[])
        n163 = flat-sequence {
          tunnel: w315 -> [w327]
          tunnel: [w326] -> w314
          tunnel: w313 -> [w326]
          tunnel: [w325] -> w312
          tunnel: w314 -> [w333]
          tunnel: w312 -> [w332]
          tunnel: [w332] -> w311
          tunnel: [w331] -> w310
          frame #0 {
            n164 = for {
              tunnel: w327 -> [w330] mode=indexing
              tunnel: [w328] -> w325 mode=indexing
              n165 = call <vilib>:"DAQmx Stop Task.vi"("task/channels in"=w330) -> ("task out"=w328:refnum<k21>)  [unwired: 13 in, 1 out]
              n166 = Wait (ms)(milliseconds to wait=u32 50) -> ()  [unwired: 1 out]
            }
          }
          frame #1 {
            n167 = for {
              tunnel: w333 -> [w336] mode=indexing
              tunnel: [w334] -> w331 mode=indexing
              n168 = call <vilib>:"DAQmx Stop Task.vi"("task/channels in"=w336) -> ("task out"=w334:refnum<k21>)  [unwired: 13 in, 1 out]
              n169 = Wait (ms)(milliseconds to wait=u32 50) -> ()  [unwired: 1 out]
            }
          }
        }
        n170 = flat-sequence {
          tunnel: w311 -> [w319]
          tunnel: w310 -> [w318]
          tunnel: [w318] -> w309
          tunnel: w309 -> [w322]
          frame #0 {
            n171 = for {
              tunnel: w319 -> [w321] mode=indexing
              n172 = Wait (ms)(milliseconds to wait=u32 50) -> ()  [unwired: 1 out]
              n173 = call <vilib>:"DAQmx Clear Task.vi"("task in"=w321) -> ()  [unwired: 14 in, 1 out]
            }
          }
          frame #1 {
            n174 = for {
              tunnel: w322 -> [w324] mode=indexing
              n175 = call <vilib>:"DAQmx Clear Task.vi"("task in"=w324) -> ()  [unwired: 14 in, 1 out]
              n176 = Wait (ms)(milliseconds to wait=u32 50) -> ()  [unwired: 1 out]
            }
          }
        }
      }
      frame 5 {
        # "This code stops AI/AO tasks, deletes them, and restarts program execution."
        n177 = local read "AO Task"() -> (w343:refnum<k21>[])
        n178 = local read "AI task"() -> (w344:refnum<k21>[])
        n179 = flat-sequence {
          tunnel: w344 -> [w351]
          tunnel: [w350] -> w346
          tunnel: w343 -> [w350]
          tunnel: [w349] -> w345
          tunnel: w346 -> [w357]
          tunnel: w345 -> [w356]
          tunnel: [w356] -> w342
          tunnel: [w355] -> w341
          tunnel: w342 -> [w361]
          tunnel: w341 -> [w362]
          tunnel: [w362] -> w340
          tunnel: w340 -> [w365]
          frame #0 {
            n180 = for {
              tunnel: w351 -> [w354] mode=indexing
              tunnel: [w352] -> w349 mode=indexing
              n181 = Wait (ms)(milliseconds to wait=u32 50) -> ()  [unwired: 1 out]
              n182 = call <vilib>:"DAQmx Stop Task.vi"("task/channels in"=w354) -> ("task out"=w352:refnum<k21>)  [unwired: 13 in, 1 out]
            }
          }
          frame #1 {
            n183 = for {
              tunnel: w357 -> [w360] mode=indexing
              tunnel: [w358] -> w355 mode=indexing
              n184 = Wait (ms)(milliseconds to wait=u32 50) -> ()  [unwired: 1 out]
              n185 = call <vilib>:"DAQmx Stop Task.vi"("task/channels in"=w360) -> ("task out"=w358:refnum<k21>)  [unwired: 13 in, 1 out]
            }
          }
          frame #2 {
            n186 = for {
              tunnel: w361 -> [w364] mode=indexing
              n187 = call <vilib>:"DAQmx Clear Task.vi"("task in"=w364) -> ()  [unwired: 14 in, 1 out]
              n188 = Wait (ms)(milliseconds to wait=u32 50) -> ()  [unwired: 1 out]
            }
          }
          frame #3 {
            n189 = for {
              tunnel: w365 -> [w367] mode=indexing
              n190 = call <vilib>:"DAQmx Clear Task.vi"("task in"=w367) -> ()  [unwired: 14 in, 1 out]
              n191 = Wait (ms)(milliseconds to wait=u32 50) -> ()  [unwired: 1 out]
            }
          }
        }
      }
    }
  }
